vi "convert_string_to_double.vi"(3 "default (0)":dbl, 4 "String in":string) -> (1 "double value out":dbl)   [LabVIEW 2022 SP3, in "hmp4000_rsidr_core.lvlib"]
uses:
  hmp4000_rsidr_core.lvlib
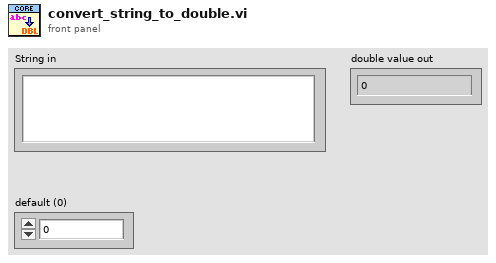
[diagram p1: front panel]
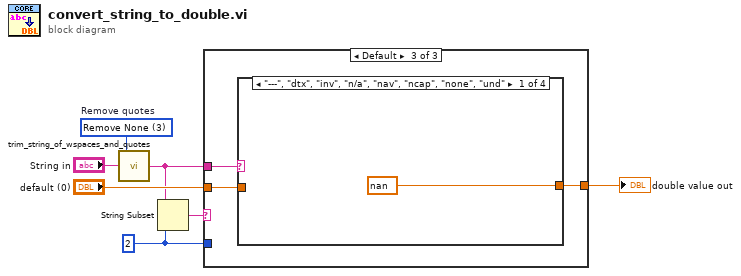
[diagram p0: block diagram]
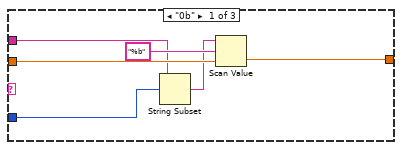
[diagram p2: hidden frame]
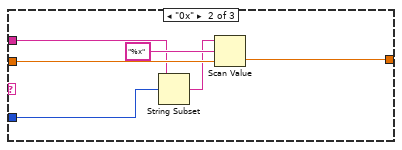
[diagram p3: hidden frame]
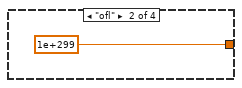
[diagram p4: hidden frame]
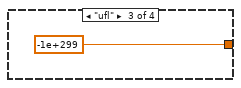
[diagram p5: hidden frame]
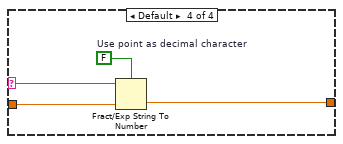
[diagram p6: hidden frame]
diagram:
  w3 = u16 3 items=["Remove All Quotes", "Remove Single Quotes", "Remove Double Quotes", "Remove None"]  # Remove quotes
  w6 = 2 ("length (rest)")
  n1 = call "trim_string_of_wspaces_and_quotes.vi"("String in"="String in", "Remove quotes (Remove All)"=w3) -> ("String out"=w1:string)  [unwired: 3 in]
  n2 = String Subset(string=w1, length (rest)=w6) -> (substring=w7:string)  [unwired: 1 in]
  n3 = case shown="Default" w7 {
    tunnel: [w13 w19 w21] -> w4
    tunnel: w1 -> [w9 w15 w20]
    tunnel: "default (0)" -> [w12 w18 w22]
    tunnel: w6 -> [w10 w16 _]
    frame "0b" {
      n4 = String Subset(string=w9, offset (0)=w10) -> (substring=w8:string)  [unwired: 1 in]
      n5 = Scan Value(string=w8, format string="%b", default (0 dbl)=w12) -> (value=w13:dbl)  [unwired: 1 out]
    }
    frame "0x" {
      n6 = String Subset(string=w15, offset (0)=w16) -> (substring=w14:string)  [unwired: 1 in]
      n7 = Scan Value(string=w14, format string="%x", default (0 dbl)=w18) -> (value=w19:dbl)  [unwired: 1 out]
    }
    frame Default {
      n8 = case shown="\"---\", \"dtx\", \"inv\", \"n/a\", \"nav\", \"ncap\", \"none\", \"und\"" w20 {
        selector: w20 -> [_ _ _ w26]
        tunnel: w22 -> [_ _ _ w29]
        tunnel: [nan 1e+299 -1e+299 w28] -> w21
        frame "---", "dtx", "inv", "n/a", "nav", "ncap", "none", "und" {
        }
        frame "ofl" {
        }
        frame "ufl" {
        }
        frame Default {
          w27 = FALSE  # Use point as decimal character
          n9 = Fract/Exp String To Number(use system decimal point (T)=w27, string=w26, default (0 dbl)=w29) -> (number=w28:dbl)  [unwired: 1 in, 1 out]
        }
      }
    }
  }
  "double value out" <- w4
